vi "Emballage_BDD_scan1Valve.vi"(8 "Error in":errorcluster caption="Error in (no error)", 11 "Instruction_IN":string="Veuillez scanner le bloc/la valve \nà enlever/remplacer!") -> (0 "Error out":errorcluster, 2 "TIMEOUT_FIN?":bool, 3 "produit scanné:":string)   [LabVIEW 2020]
uses:
  enum_ON_OFF_Lecteur.ctl
  Modules/FS/60_FS_Controles/60_FS_SetGet.ctl
panel:
  out "Instruction":string
  # "Veuillez scanner le bloc/la valve \nà enlever/remplacer!"
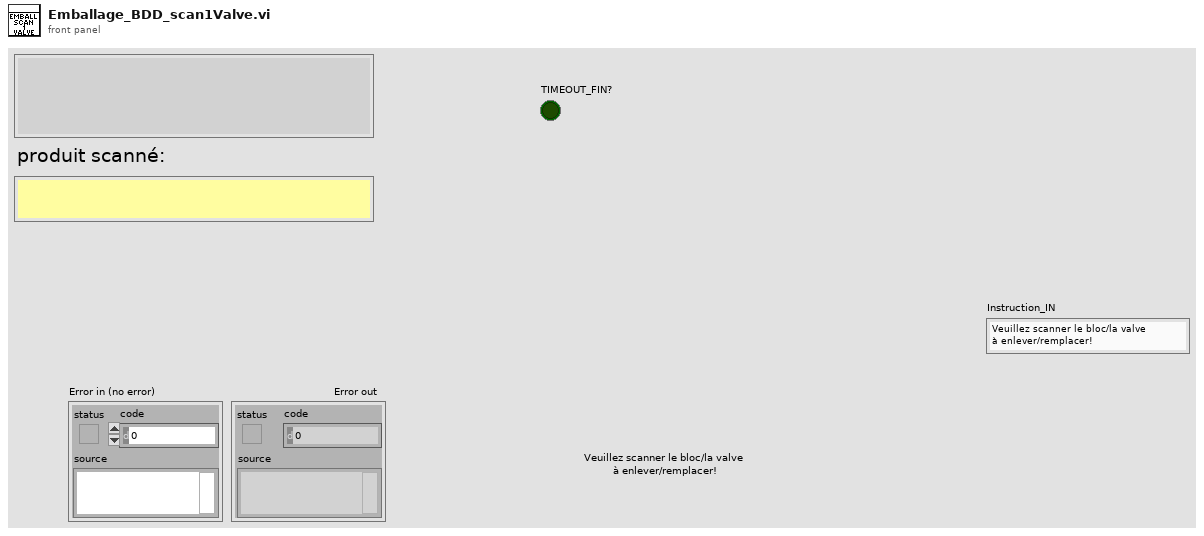
[diagram p1: front panel]
types:
  T1 = typedef "enum_ON_OFF_Lecteur.ctl" = enum16{"ON_COURT", "OFF", "ON", "OFF (open/Close)", "ON (open/close)"}
  T2 = typedef "60_FS_SetGet.ctl" = enum16{"set", "get"}
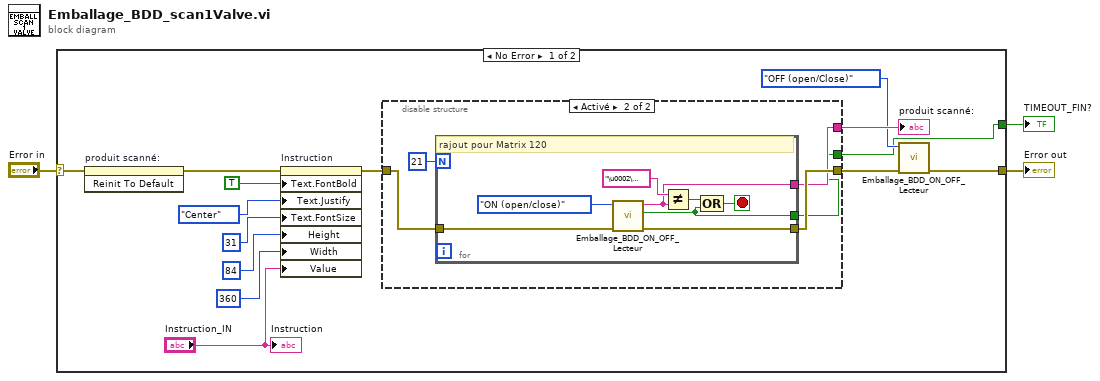
[diagram p0: block diagram]
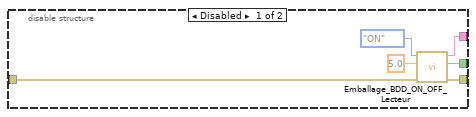
[diagram p2: hidden frame]
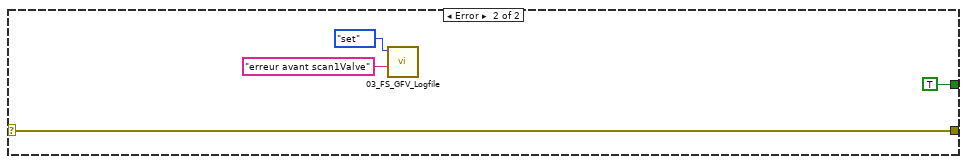
[diagram p3: hidden frame]
diagram:
  n1 = case shown="No Error" "Error in" {
    selector: "Error in" -> [w10 w40]
    tunnel: [w5 w40] -> w2
    tunnel: [w4 TRUE ("status")] -> w1
    frame No Error {
      n2 = invoke on="produit scanné:" class="Ch" method="Reinit To Default"(error in=w10) -> (error out=w12:errorcluster)  [unwired: 2 in, 2 out]
      n3 = property on="Instruction" class="Str"(error in=w12, "Text.FontBold"=TRUE ("Texte.Police:Gras"), "Text.Justify"=enum16{"Left", "Center", "Right"}."Center" ("Texte.Justification"), "Text.FontSize"=u32 31 ("Texte.Taille:Hauteur"), "Height"=u32 84 ("Taille:Hauteur"), "Width"=u32 360 ("Taille:Largeur"), "Value"="Instruction_IN") -> (error out=w9:errorcluster)  [unwired: 1 in, 1 out]
      n4 = disable-structure shown="Activé" {
        disable-tunnel: w9 -> [w22 w28]
        disable-tunnel: [w21 w26] -> w8
        disable-tunnel: [w20 w27] -> w6
        disable-tunnel: [w19 w25] -> w4
        frame Disabled {
          n5 = call "Emballage_BDD_ON_OFF_Lecteur.vi"("Error in"=w22, "TimeOut (sec)"=5.0, "ON/OFF lecteur"=enum_ON_OFF_Lecteur."ON") -> ("Error out"=w20:errorcluster, "TIMEOUT_FIN?"=w19:bool, "Etiquette scanné"=w21:string)  [unwired: 6 in]
        }
        frame Enabled {
          n6 = for {
            N: 21 -> [_]
            tunnel: [w30] -> w26
            tunnel: [w32] -> w25
            tunnel: w28 -> [w36]
            tunnel: [w34] -> w27
            stop <- w33 stop-if-true
            # "rajout pour Matrix 120"
            n7 = call "Emballage_BDD_ON_OFF_Lecteur.vi"("Error in"=w36, "ON/OFF lecteur"=enum_ON_OFF_Lecteur."ON (open/close)") -> ("Error out"=w34:errorcluster, "TIMEOUT_FIN?"=w32:bool, "Etiquette scanné"=w30:string)  [unwired: 7 in]
            n8 = Not Equal?(x="\u0002\u0018", y=w30) -> (x != y?=w29:bool)
            n9 = Compound Arithmetic op=OR ("Opérateur arithmétique")(w29, w32) -> (w33:bool)
          }
        }
      }
      "produit scanné:" <- w8
      n10 = call "Emballage_BDD_ON_OFF_Lecteur.vi"("Error in"=w6, "ON/OFF lecteur"=enum_ON_OFF_Lecteur."OFF (open/Close)") -> ("Error out"=w5:errorcluster)  [unwired: 7 in, 2 out]
      "Instruction" <- "Instruction_IN"
    }
    frame Error {
      n11 = call "03_FS_GFV_Logfile.vi"("Chaîne"="erreur avant scan1Valve", "States"=60_FS_SetGet."set") -> ()  [unwired: 8 in, 2 out]
    }
  }
  "Error out" <- w2
  "TIMEOUT_FIN?" <- w1
